vi "Close.vi"(6 "Update name":bool, 7 "Delay":u32=10 format="%.0fms", 8 "error in (no error)":errorcluster, 9 "Time Stamp":timestamp, 10 "Clean up":bool=TRUE, 11 "File in":refnum<class "File.lvclass">) -> (0 "error out":errorcluster, 1 "Actually closed":bool, 2 "File Path":path, 3 "File out":refnum<class "File.lvclass">)   [LabVIEW 2024, in "File.lvclass"]
uses:
  File.lvclass
  File.lvclass/File.ctl
  Read Is open.vi
  Read tdms stream.vi
  Write tdms stream.vi
  Write Is open.vi
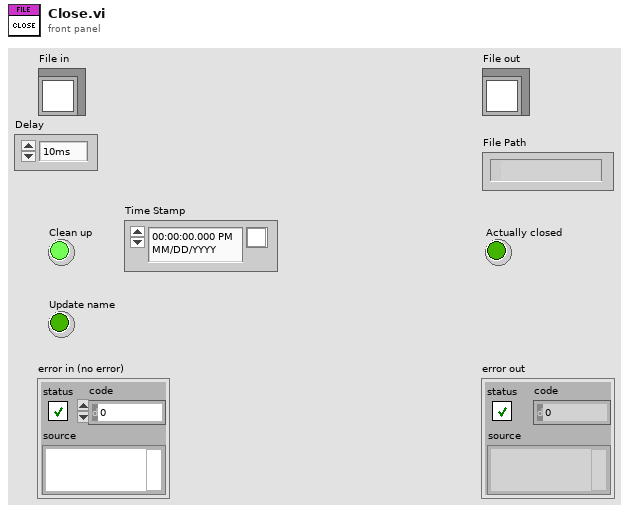
[diagram p1: front panel]
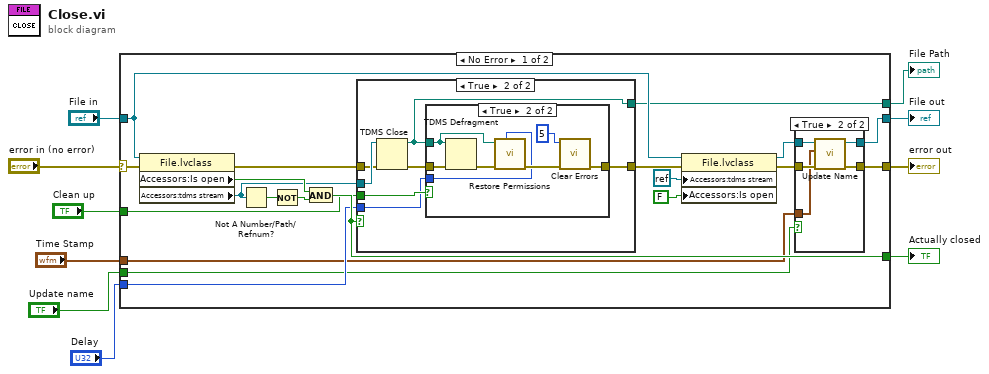
[diagram p0: block diagram]
diagram:
  n1 = case shown="No Error" "error in (no error)" {
    selector: "error in (no error)" -> [w25 w55]
    tunnel: [w12 w55] -> w9
    tunnel: [w13 w54] -> w7
    tunnel: "File in" -> [w24 w54]
    tunnel: [w20 _] -> w6
    tunnel: [w19 _] -> w5
    tunnel: "Clean up" -> [w18 _]
    tunnel: "Delay" -> [w17 _]
    tunnel: "Update name" -> [w16 _]
    tunnel: "Time Stamp" -> [w11 _]
    frame No Error {
      n2 = property class="File.lvclass"(reference=w24, error in=w25) -> (error out=w30:errorcluster, "Accessors:Is open"=w29:bool, "Accessors:tdms stream"=w28:refnum<k34>)  [unwired: 1 out]
      n3 = Not A Number/Path/Refnum?(number/path/refnum=w28) -> (NaN/Path/Refnum?=w27:bool)
      n4 = Not(x=w27) -> (.not. x?=w26:bool)
      n5 = And(x=w29, y=w26) -> (x .and. y?=w20:bool)
      n6 = case shown="True" w20 {
        tunnel: w30 -> [w38 w44]
        tunnel: w28 -> [_ w45]
        tunnel: [w38 w40] -> w21
        tunnel: [_ w42] -> w19
        tunnel: w18 -> [_ w43]
        tunnel: w17 -> [_ w39]
        frame False {
        }
        frame True {
          n7 = TDMS Close(8:w44, 11:w45) -> (0:w41:errorcluster, 3:w42:path)
          n8 = case shown="True" w43 {
            tunnel: w42 -> [_ w48]
            tunnel: w41 -> [w46 w50]
            tunnel: [w46 w49] -> w40
            tunnel: w39 -> [_ w47]
            frame False {
            }
            frame True {
              n9 = TDMS Defragment(4:w50, 7:w48) -> (0:w51:errorcluster)
              n10 = call "Restore Permissions.vi"("Delay"=w47, "Error In"=w51, "File Path"=w48) -> ("Error Out"=w53:errorcluster)  [unwired: 5 in, 3 out]
              n11 = call <vilib>:"Clear Errors.vi"("error in (no error)"=w53, "specific error code to clear (0: all)"=5) -> ("error out"=w49:errorcluster)  [unwired: 4 in, 1 out]
            }
          }
        }
      }
      n12 = property class="File.lvclass"(reference=w24, error in=w21, "Accessors:tdms stream"=refnum<k0> refnum, "Accessors:Is open"=FALSE ("Is open")) -> (reference out=w14:refnum<class "File.lvclass">, error out=w15:errorcluster)
      n13 = case shown="True" w16 {
        tunnel: w15 -> [w32 w37]
        tunnel: w14 -> [w31 w36]
        tunnel: [w31 w35] -> w13
        tunnel: [w32 w34] -> w12
        tunnel: w11 -> [_ w33]
        frame False {
        }
        frame True {
          n14 = call-dynamic "Update Name.vi"("error in (no error)"=w37, "Time Stamp"=w33, "File in"=w36) -> ("error out"=w34:errorcluster, "File out"=w35:refnum<class "File.lvclass">)  [unwired: 7 in]
        }
      }
    }
    frame Error {
    }
  }
  "error out" <- w9
  "File out" <- w7
  "Actually closed" <- w6
  "File Path" <- w5
